vi "Configure Infiniimode.vi"(8 "error in (no error)":errorcluster, 9 "Infinii Mode (0: Differential)":i32(ring) items=["Differential", "SEA", "SEB", "CM"], 10 "Channel (1: Channel 1)":i32(ring)=1 items=["Channel 1"=1, "Channel 2"=2, "Channel 3"=3, "Channel 4"=4], 11 "VISA resource name":refnum<visa-resource-name>) -> (0 "error out":errorcluster, 3 "VISA resource name out":refnum<visa-resource-name>)   [LabVIEW 2020, in "Agilent 90000 Series.lvlib"]
doc: "Configures the N2750A probe's InfiniiMode."
uses:
  Agilent 90000 Series.lvlib
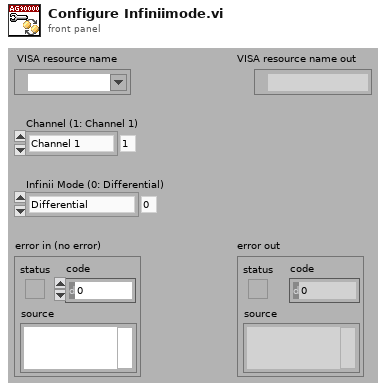
[diagram p1: front panel]
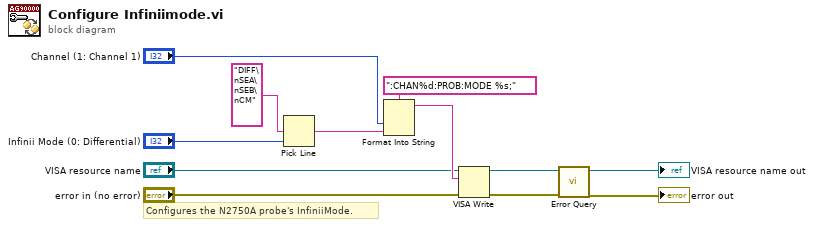
[diagram p0: block diagram]
diagram:
  # "Configures the N2750A probe's InfiniiMode."
  n1 = Pick Line(multi-line string="DIFF\nSEA\nSEB\nCM", line index="Infinii Mode (0: Differential)") -> (output string=w8:string)  [unwired: 1 out]
  n2 = Format Into String(format string=":CHAN%d:PROB:MODE %s;", "Channel (1: Channel 1)", w8) -> (resulting string=w7:string)  [unwired: 2 in, 1 out]
  n3 = VISA Write(VISA resource name="VISA resource name", write buffer=w7, error in (no error)="error in (no error)") -> (VISA resource name out=w4:refnum<visa-resource-name>, error out=w3:errorcluster)  [unwired: 1 out]
  n4 = call "Error Query.vi"("error in (no error)"=w3, "VISA resource name"=w4) -> ("error out"=→"error out":errorcluster, "VISA resource name out"=→"VISA resource name out":refnum<visa-resource-name>)  [unwired: 8 out]
